vi "IS Documentation.vi"   [LabVIEW 2017]
uses:
  Data Helpers/IS PolyVI Instance String to JSON Cluster.vi
  IS PolyVI Instance DBL To JSON Cluster .vi
  Data Helpers/IS PolyVI Instance Bool To JSON Cluster .vi
panel:
  # "GO TO BLOCK DIAGRAM!"
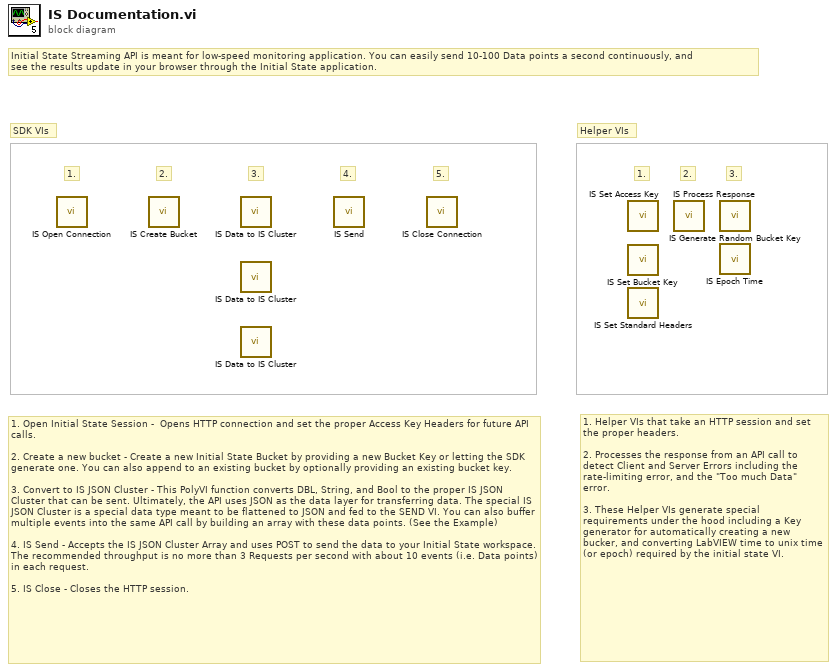
[diagram p0: block diagram]
diagram:
  # "1. Helper VIs that take an HTTP session and set the proper headers. \n\n2. Processes the response from an API call to detect Client and Server Errors including the rate-limiting error, and the \"Too much Data\" error.\n\n3. These Helper VIs generate special requirements under the hood including a Key generator for automatically creating a new bucker, and converting LabVIEW time to unix time (or epoch) required by the initial state VI."
  # "Initial State Streaming API is meant for low-speed monitoring application. You can easily send 10-100 Data points a second continuously, and \nsee the results update in your browser through the Initial State application."
  # "1. Open Initial State Session -  Opens HTTP connection and set the proper Access Key Headers for future API calls. \n\n2. Create a new bucket - Create a new Initial State Bucket by providing a new Bucket Key or letting the SDK generate one. You can also append to an existing bucket by optionally providing an existing bucket key. \n\n3. Convert to IS JSON Cluster - This PolyVI function converts DBL, String, and Bool to the proper IS JSON Cluster that can be sent. Ultimately, the API uses JSON as the data layer for transferring data. The special IS JSON Cluster is a special data type meant to be flattened to JSON and fed to the SEND VI. You can also buffer multiple events into the same API call by building an array with these data points. (See the Example)\n\n4. IS Send - Accepts the IS JSON Cluster Array and uses POST to send the data to your Initial State workspace. The recommended throughput is no more than 3 Requests per second with about 10 events (i.e. Data points) in each request. \n\n5. IS Close - Closes the HTTP session."
  # "3."
  # "2."
  # "1."
  # "5."
  # "4."
  # "3."
  # "2."
  # "1."
  # "Helper VIs"
  # "SDK VIs"
  n1 = call "IS Open Connection.vi"() -> ()  [unwired: 10 in, 2 out]
  n2 = call "IS Create Bucket.vi"() -> ()  [unwired: 9 in, 3 out]
  n3 = call-poly "IS Data to IS Cluster.vi"() -> ()  [unwired: 5 in, 1 out]
  n4 = call-poly "IS Data to IS Cluster.vi"() -> ()  [unwired: 5 in, 1 out]
  n5 = call-poly "IS Data to IS Cluster.vi"() -> ()  [unwired: 5 in, 1 out]
  n6 = call "IS Send.vi"() -> ()  [unwired: 6 in, 6 out]
  n7 = call "IS Close Connection.vi"() -> ()  [unwired: 11 in, 1 out]
  n8 = call "IS Set Access Key.vi"() -> ()  [unwired: 9 in, 2 out]
  n9 = call "IS Set Bucket Key.vi"() -> ()  [unwired: 9 in, 2 out]
  n10 = call "IS Set Standard Headers.vi"() -> ()  [unwired: 10 in, 2 out]
  n11 = call "IS Process Response.vi"() -> ()  [unwired: 10 in, 2 out]
  n12 = call "IS Generate Random Bucket Key.vi"() -> ()  [unwired: 11 in, 1 out]
  n13 = call "IS Epoch Time.vi"() -> ()  [unwired: 11 in, 1 out]
